vi "frontpanel.vi"() -> ()   [LabVIEW 2019]
panel:
  out "Boolean 3":bool
  out "Boolean 2":bool
  in  "Numeric Control":dbl
  in  "Boolean":bool
  out "Gauge":dbl(knob) scale=0.0..10.0
  in  "Vertical Fill Slide":dbl(slide) scale=0.0..10.0
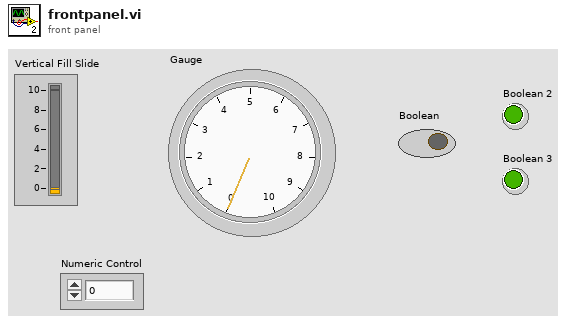
[diagram p1: front panel]
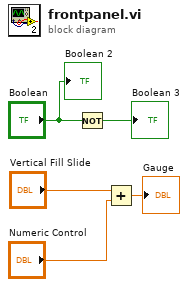
[diagram p0: block diagram]
diagram:
  n1 = Not(x="Boolean") -> (.not. x?=→"Boolean 3":bool)
  n2 = Add(x="Vertical Fill Slide", y="Numeric Control") -> (x+y=→"Gauge":dbl)
  "Boolean 2" <- "Boolean"
